vi "Simple.vi"() -> ()   [LabVIEW 2014]
uses:
  Public/Controls/Severity.ctl
  Public/Controls/Configuration.ctl
  CF-Logger.lvlib
panel:
  out "Messages":i32(listbox)
  in  "Stop":bool
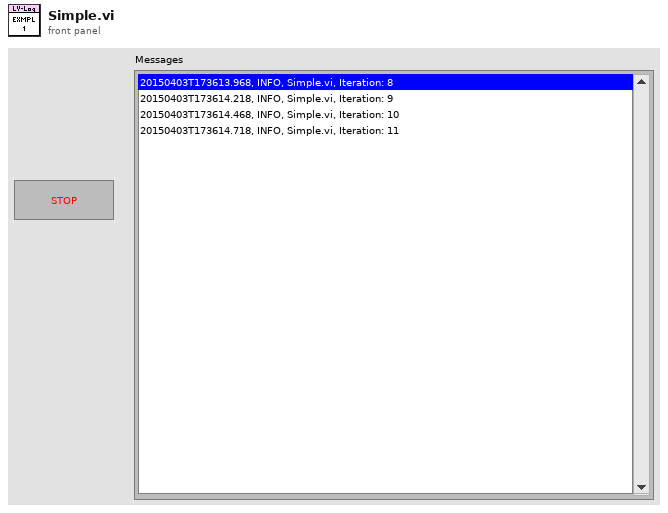
[diagram p1: front panel]
types:
  T1 = typedef "CF-Logger.lvlib/Configuration.ctl" = cluster{"Root Folder":path, "File Size Limit":i64, "Application Name":string}
  T2 = typedef "CF-Logger.lvlib/Severity.ctl" = enum16{"Benign", "Warning", "Recoverable", "Fatal"}
  T3 = typedef "LV-Logger.lvlib/Message.ctl" = cluster{"Time Stamp":timestamp, "Tag":T4, "Source":string, "Text":string}
  T4 = typedef "LV-Logger.lvlib/Tag.ctl" = enum16{"Fatal", "Error", "Warn", "Info", "Debug", "Trace"}
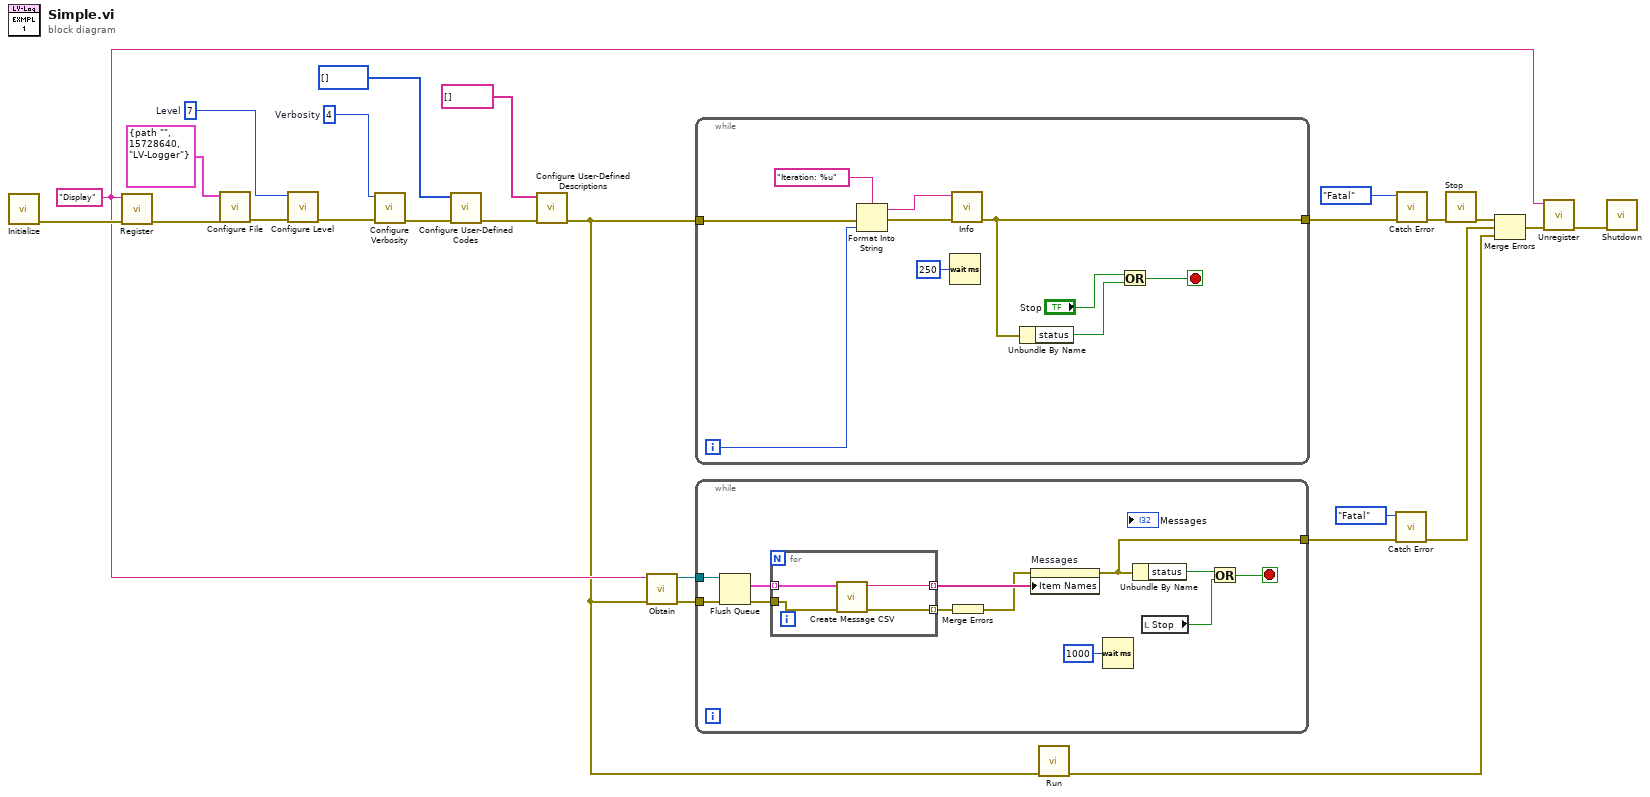
[diagram p0: block diagram]
diagram:
  w9 = u8 7  # Level
  w6 = u8 4  # Verbosity
  w19 = "Display" ("Listener ID")
  n1 = call "Initialize.vi"() -> ("Error Out"=w25:errorcluster)  [unwired: 11 in]
  n2 = call "Register.vi"("Error In"=w25, "Listener ID"=w19) -> ("Error Out"=w11:errorcluster)  [unwired: 9 in]
  n3 = call "Configure File.vi"("Error In"=w11, "Configuration"=T1 {"Root Folder"=path "", "File Size Limit"=15728640, "Application Name"="LV-Logger"}) -> ("Error Out"=w8:errorcluster)  [unwired: 9 in]
  n4 = call "Configure Level.vi"("Error In"=w8, "Level"=w9) -> ("Error Out"=w7:errorcluster)  [unwired: 9 in]
  n5 = call "Configure Verbosity.vi"("Error In"=w7, "Verbosity"=w6) -> ("Error Out"=w5:errorcluster)  [unwired: 9 in]
  n6 = call "Configure User-Defined Codes.vi"("Error In"=w5, "User-Defined Codes"=i32[] []) -> ("Error Out"=w3:errorcluster)  [unwired: 9 in]
  n7 = call "Configure User-Defined Descriptions.vi"("Error In"=w3, "User-Defined Descriptions"=string[] []) -> ("Error Out"=w1:errorcluster)  [unwired: 9 in]
  n8 = call "Obtain.vi"("Error In"=w1, "Listener ID"=w19) -> ("Error Out"=w22:errorcluster, "Listener"=w23:refnum<queue>)  [unwired: 8 in]
  n9 = while {
    tunnel: [w27] -> w17
    tunnel: w1 -> [w26]
    i -> [w35]
    stop <- w31 stop-if-true
    n10 = Format Into String(format string="Iteration: %u", error in=w26, w35) -> (resulting string=w30:string, error out=w33:errorcluster)  [unwired: 1 in]
    n11 = Wait (ms)(milliseconds to wait=u32 250) -> ()  [unwired: 1 out]
    n12 = call "Info.vi"("Error In"=w33, "Text"=w30) -> ("Error Out"=w27:errorcluster)  [unwired: 9 in]
    n13 = Unbundle By Name(w27) -> ("status"=w28:bool)
    n14 = Or(x="Stop", y=w28) -> (x .or. y?=w31:bool)
  }
  n15 = while {
    tunnel: w23 -> [w47]
    tunnel: w22 -> [w46]
    tunnel: [w36] -> w21
    stop <- w38 stop-if-true
    n16 = Flush Queue(queue=w47, error in (no error)=w46) -> (remaining elements=w45:T3[], error out=w44:errorcluster)  [unwired: 1 out]
    n17 = for {
      tunnel: w45 -> [w51] mode=indexing
      tunnel: w44 -> [w50]
      tunnel: [w49] -> w43 mode=indexing
      tunnel: [w48] -> w42 mode=indexing
      n18 = call "Create Message CSV.vi"("Error In"=w50, "Message"=w51) -> ("Error Out"=w48:errorcluster, "CSV"=w49:string)  [unwired: 8 in]
    }
    n19 = Merge Errors(w42) -> (w41:errorcluster)
    n20 = property on="Messages" class="LstBox (strict)"(error in=w41, "Item Names"=w43) -> (error out=w36:errorcluster)  [unwired: 1 in, 1 out]
    n21 = Wait (ms)(milliseconds to wait=u32 1000) -> ()  [unwired: 1 out]
    n22 = Unbundle By Name(w36) -> ("status"=w40:bool)
    n23 = local read "Stop"() -> (w39:bool)
    n24 = Or(x=w40, y=w39) -> (x .or. y?=w38:bool)
  }
  n25 = call "Run.vi"("Error In"=w1) -> ("Error Out"=w18:errorcluster)  [unwired: 10 in]
  n26 = call "Catch Error.vi"("Error In"=w21, "Severity"=Severity."Fatal") -> ("Error Out"=w13:errorcluster)  [unwired: 9 in]
  n27 = call "Catch Error.vi"("Error In"=w17, "Severity"=Severity."Fatal") -> ("Error Out"=w15:errorcluster)  [unwired: 9 in]
  n28 = call "Stop.vi"("Error In"=w15) -> ("Error Out"=w16:errorcluster)  [unwired: 10 in]
  n29 = Merge Errors(w16, w13, w18) -> (w20:errorcluster)
  n30 = call "Unregister.vi"("Error In"=w20, "Listener ID"=w19) -> ("Error Out"=w24:errorcluster)  [unwired: 9 in]
  n31 = call "Shutdown.vi"("Error In"=w24) -> ()  [unwired: 10 in, 1 out]
